vi "Data_translation_example.vi"() -> ()   [LabVIEW 2010]
uses:
  National Instruments/LabVIEW 8.6/user.lib/LV-LINK/PolySubVIs/CreateAinChan.vi
  National Instruments/LabVIEW 8.6/user.lib/LV-LINK/PolySubVIs/OLTimingSetInput.vi
  National Instruments/LabVIEW 8.6/user.lib/LV-LINK/PolySubVIs/OLReadMultiple2D.vi
panel:
  out "Acquired Data 2":dbl[](graph) caption="Acquired Data"
  out "Acquired Data":dbl[][](graph)
  in  "Samples Per Channel":dbl=1000.0
  in  "Sample Rate":dbl=10000.0
  in  "?":bool
  in  "Channels":string="Ain 0"
  # "Continuous Analog Input Example"
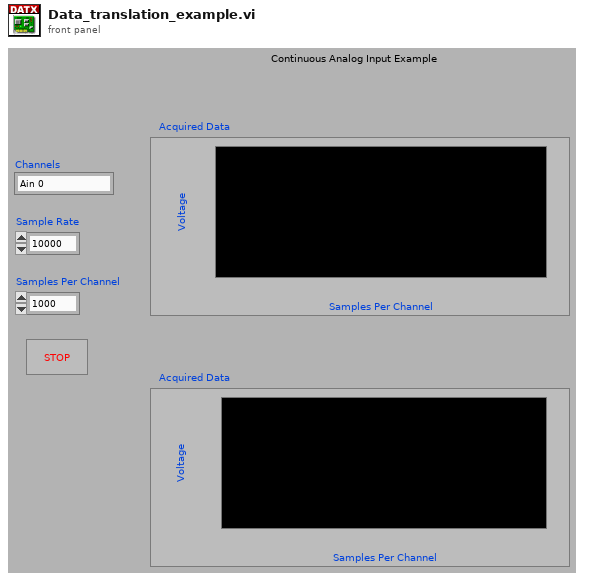
[diagram p1: front panel]
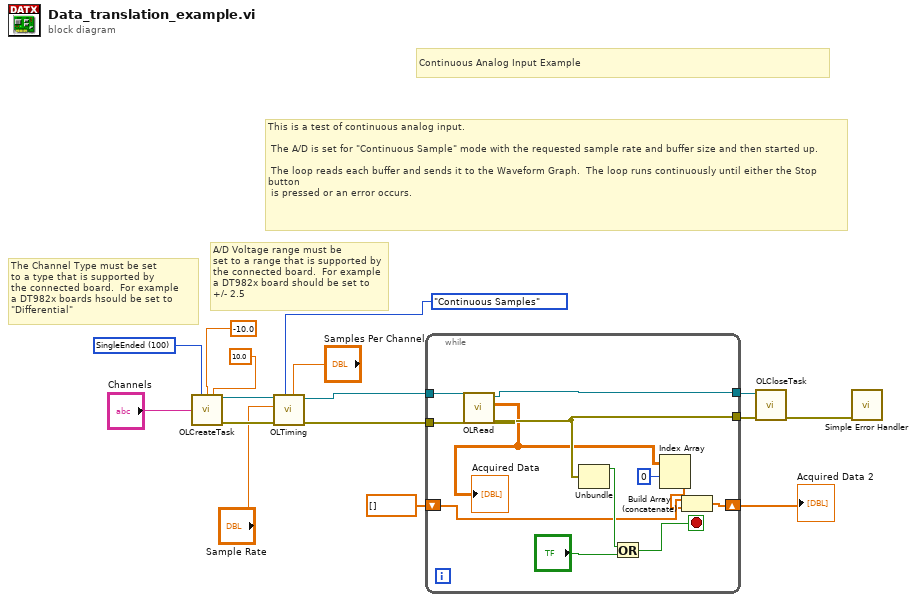
[diagram p0: block diagram]
diagram:
  w6 = 100 items=["SingleEnded"=100, "Differential"=101] ("Channel Type")
  # "The Channel Type must be set\nto a type that is supported by \nthe connected board.  For example\na DT982x boards hsould be set to\n\"Differential\""
  # "A/D Voltage range must be\nset to a range that is supported by \nthe connected board.  For example\na DT982x board should be set to \n+/- 2.5"
  # "Continuous Analog Input Example"
  # "This is a test of continuous analog input. \n\n The A/D is set for \"Continuous Sample\" mode with the requested sample rate and buffer size and then started up.\n\n The loop reads each buffer and sends it to the Waveform Graph.  The loop runs continuously until either the Stop button\n is pressed or an error occurs."
  n1 = call-poly "OLCreateTask.vi"("Channel Type"=w6, "Range Min"=-10.0, "Range Max"=10.0, "Channel"="Channels") -> ("Task Out"=w4:refnum<k24>, "error out"=w15:errorcluster)  [unwired: 10 in]
  n2 = call-poly "OLTiming.vi"("Samples Per Channel"="Samples Per Channel", "Sample Mode"=enum16{"Finite Samples", "Continuous Samples"}."Continuous Samples", "error in (no error)"=w15, "Sample Freq (Hz)"="Sample Rate", "Task In"=w4) -> ("error out"=w7:errorcluster, "Task Out"=w8:refnum<k24>)  [unwired: 4 in, 1 out]
  n3 = while {
    tunnel: w7 -> [w28]
    tunnel: [w27] -> w10
    tunnel: [w26] -> w9
    tunnel: w8 -> [w23]
    shift-right: [w19] -> w1
    shift-left: dbl[] [] -> [w18]
    stop <- w22 stop-if-true
    n4 = call-poly "OLRead.vi"("error in (no error)"=w28, "Task In"=w23) -> ("error out"=w26:errorcluster, "ReadData"=w21:dbl[][], "Task Out"=w27:refnum<k24>)  [unwired: 7 in]
    "Acquired Data" <- w21
    n5 = Unbundle(w26) -> ("status"=w25:bool)  [unwired: 2 out]
    n6 = Or(x=w25, y="?") -> (x .or. y?=w22:bool)
    n7 = Index Array(array=w21, index (row)=0) -> (element=w17:dbl[])  [unwired: 1 in]
    n8 = Build Array (concatenate)(w18, w17) -> (w19:dbl[])
  }
  "Acquired Data 2" <- w1
  n9 = call "OLCloseTask.vi"("Error in"=w9, "Task In"=w10) -> ("Error Out"=w12:errorcluster)  [unwired: 9 in]
  n10 = call <vilib>:"Simple Error Handler.vi"("error in (no error)"=w12) -> ()  [unwired: 4 in, 5 out]
